vi "Initialize HW.vi"(8 "error in (no error)":errorcluster, 11 "DAQmx Force Sensor in":refnum<class "DAQmx Force Sensor.lvclass">) -> (0 "error out":errorcluster, 3 "DAQmx Force Sensor out":refnum<class "DAQmx Force Sensor.lvclass">)   [LabVIEW 2020, in "DAQmx Force Sensor.lvclass"]
uses:
  DAQmx Force Sensor.lvclass
  C:/Users/jharw/Documents/1 Folder to Rule them All/UMD/Inflation-Apparatus/src/Hardware/General Hardware.lvclass
  General Hardware.lvclass/General Hardware.ctl
  DAQmx Force Sensor.lvclass/DAQmx Force Sensor.ctl
  <vilib>/DAQmx/create/channels.llb/DAQmx Create Channel (AI-Voltage-Basic).vi
  <vilib>/DAQmx/configure/timing.llb/DAQmx Timing (Sample Clock).vi
  Force Sensor.lvclass
  General Hardware.lvclass
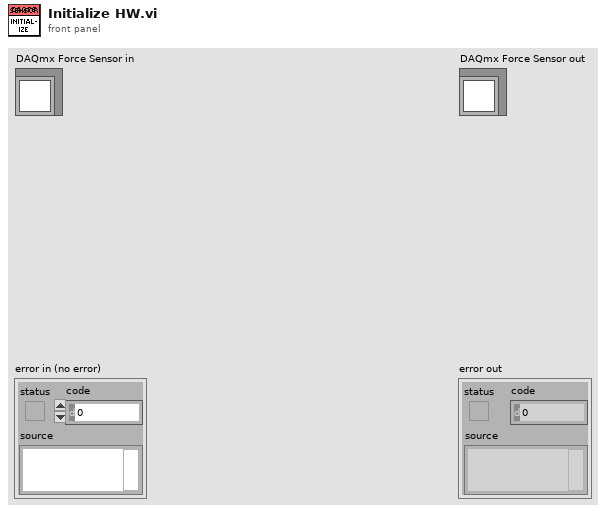
[diagram p1: front panel]
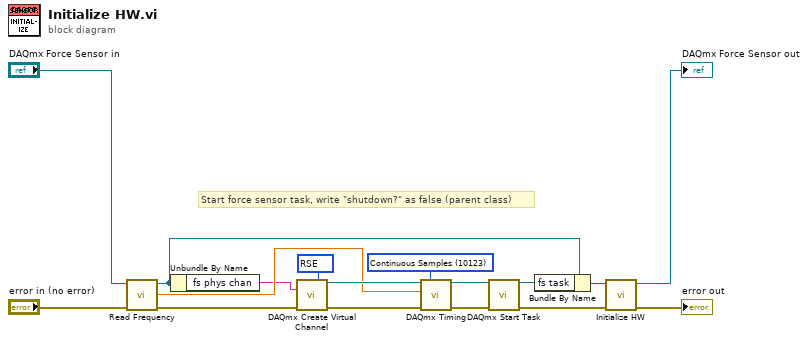
[diagram p0: block diagram]
diagram:
  w14 = 10083 items=["Default"=-1, "RSE"=10083, "NRSE"=10078, "Differential"=10106, "Pseudodifferential"=12529] ("input terminal configuration")
  w13 = 10123 items=["Finite Samples"=10178, "Continuous Samples"=10123, "Hardware Timed Single Point"=12522] ("sample mode")
  # "Start force sensor task, write \"shutdown?\" as false (parent class)"
  n1 = call "Read Frequency.vi"("error in (no error)"="error in (no error)", "General Hardware in"="DAQmx Force Sensor in") -> ("error out"=w11:errorcluster, "frequency (Hz)"=w7:dbl, "General Hardware out"=w4:refnum<class "DAQmx Force Sensor.lvclass">)  [unwired: 7 in]
  n2 = Unbundle By Name(w4) -> ("fs phys chan"=w5:tag)
  n3 = call-poly <vilib>:"DAQmx Create Virtual Channel.vi"("input terminal configuration"=w14, "physical channels"=w5, "error in"=w11) -> ("task out"=w15:refnum<k21>, "error out"=w16:errorcluster)  [unwired: 11 in]
  n4 = call-poly <vilib>:"DAQmx Timing.vi"("task/channels in"=w15, "sample mode"=w13, "rate"=w7, "error in"=w16) -> ("task out"=w8:refnum<k21>, "error out"=w10:errorcluster)  [unwired: 10 in]
  n5 = call <vilib>:"DAQmx Start Task.vi"("task/channels in"=w8, "error in"=w10) -> ("task out"=w3:refnum<k21>, "error out"=w9:errorcluster)  [unwired: 12 in]
  n6 = Bundle By Name(cluster=w4, "fs task"=w3) -> (w2:refnum<class "DAQmx Force Sensor.lvclass">)
  n7 = call-parent "Initialize HW.vi"("error in (no error)"=w9, "Force Sensor in"=w2) -> ("error out"=→"error out":errorcluster, "Force Sensor out"=→"DAQmx Force Sensor out":refnum<class "DAQmx Force Sensor.lvclass">)  [unwired: 8 in]
